vi "ConvertPathtoVSEnum.vi"(11 "Path In":path) -> (2 "Remaining Path":string, 3 "VS Enum Out":T1(ring))   [LabVIEW 2015, in "Configuration Tool.lvlib"]
uses:
  Configuration Tool.lvlib
  <vilib>/Utility/sysdir.llb/System Directory Type.ctl
  Global Settings.vi
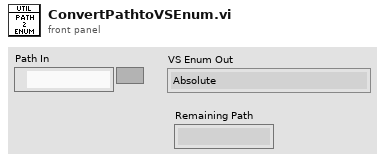
[diagram p1: front panel]
types:
  T1 = enum16{"Absolute", "To Base", "To Common Doc Dir", "To Application Data Dir"}
  T2 = typedef "System Directory Type.ctl" = i32
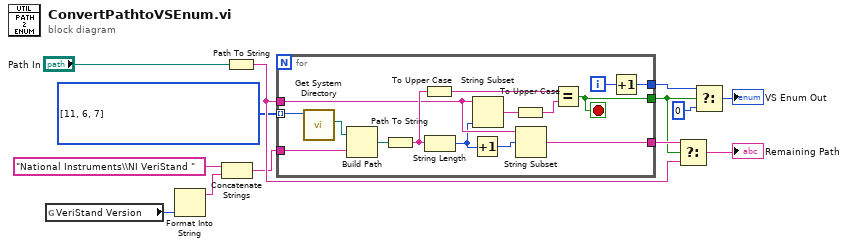
[diagram p0: block diagram]
diagram:
  w7 = T2[] [11, 6, 7] items=["User Home"=0, "User Desktop"=1, "User Documents"=2, "User Application Data"=3, "User Preferences"=4, "User Temporary"=5, "Public Documents"=6, "Public Application Data"=7, "Public Preferences"=8, "Public Cache"=13, "System Core Libraries"=9, "System Installed Libraries"=10, "Application Files"=11, "Boot Volume Root"=12]
  n1 = global read "Global Settings.vi" "VeriStand Version"() -> (w4:enum16{"2013", "2014", "2015", "2016"})
  n2 = Format Into String(w4) -> (resulting string=w3:string)  [unwired: 3 in, 1 out]
  n3 = Concatenate Strings("National Instruments\\NI VeriStand " ("name or relative path"), w3) -> (w1:string)
  n4 = Path To String(path="Path In") -> (string=w11:string)
  n5 = for {
    tunnel: w7 -> [w28] mode=indexing
    tunnel: w11 -> [w20]
    tunnel: [w26] -> w8
    tunnel: [w25] -> w10
    tunnel: [w19] -> w12
    tunnel: w1 -> [w17]
    i -> [w27]
    stop <- w25 stop-if-true
    n6 = call <vilib>:"Get System Directory.vi"("system directory type"=w28) -> ("system directory"=w18:path)  [unwired: 10 in]
    n7 = Build Path(base path=w18, name or relative path=w17) -> (appended path=w16:path)
    n8 = Path To String(path=w16) -> (string=w24:string)
    n9 = To Upper Case(1:w24) -> (0:w22:string)
    n10 = String Length(string=w24) -> (length=w14:i32)
    n11 = Increment(x=w14) -> (x+1=w15:i32)
    n12 = String Subset(string=w20, length (rest)=w14) -> (substring=w21:string)  [unwired: 1 in]
    n13 = To Upper Case(1:w21) -> (0:w23:string)
    n14 = String Subset(string=w20, offset (0)=w15) -> (substring=w19:string)  [unwired: 1 in]
    n15 = Equal?(x=w22, y=w23) -> (x = y?=w25:bool)
    n16 = Increment(x=w27) -> (x+1=w26:i32)
  }
  n17 = Select(t=w12, s=w10, f=w11) -> (s? t:f=→"Remaining Path":string)
  n18 = Select(t=w8, s=w10, f=0) -> (s? t:f=→"VS Enum Out":i32)
